vi "Create folder if not exist.vi"(8 "error in (no error) 2":errorcluster, 11 "Directory to try":string) -> (0 "error out":errorcluster, 3 "Directory Out":string)   [LabVIEW 2015]
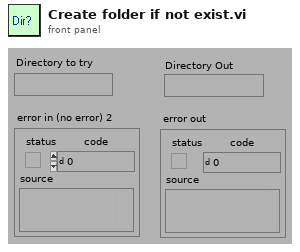
[diagram p1: front panel]
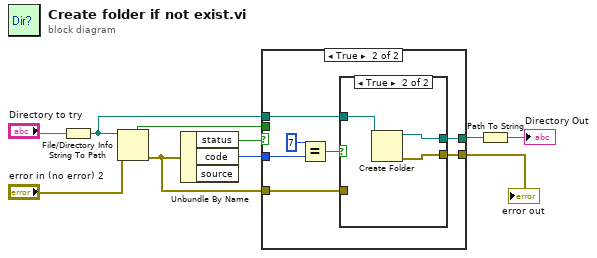
[diagram p0: block diagram]
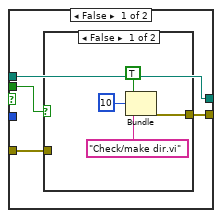
[diagram p2: hidden frame]
diagram:
  n1 = String To Path(string="Directory to try") -> (path=w7:path)
  n2 = File/Directory Info(path=w7, error in="error in (no error) 2") -> (directory=w6:bool, error out=w5:errorcluster)  [unwired: 5 out]
  n3 = Unbundle By Name(w5) -> ("status"=w8:bool, "code"=w9:i32)  [unwired: 1 out]
  n4 = case shown="True" w8 {
    tunnel: w9 -> [_ w25]
    tunnel: w7 -> [w11 w23]
    tunnel: w6 -> [w14 _]
    tunnel: w5 -> [w12 w22]
    tunnel: [w13 w21] -> w4
    tunnel: [w11 w20] -> w2
    frame False {
      n5 = case shown="False" w14 {
        tunnel: [w15 w19] -> w13
        tunnel: w12 -> [_ w19]
        frame False {
          n6 = Bundle(TRUE, 10, "Check/make dir.vi") -> (w15:errorcluster)  [unwired: 1 out]
        }
        frame True {
        }
      }
    }
    frame True {
      n7 = Equal?(x=7, y=w25) -> (x = y?=w24:bool)
      n8 = case shown="True" w24 {
        tunnel: w23 -> [w27 w31]
        tunnel: w22 -> [w28 _]
        tunnel: [w28 w30] -> w21
        tunnel: [w27 w29] -> w20
        frame False {
        }
        frame True {
          n9 = Create Folder(path (use dialog)=w31) -> (created path=w29:path, error out=w30:errorcluster)  [unwired: 1 in, 2 out]
        }
      }
    }
  }
  "error out" <- w4
  n10 = Path To String(path=w2) -> (string=→"Directory Out":string)
